vi "Scan Registry for USB Device.vi"() -> ()   [LabVIEW 2022 SP3]
uses:
  <vilib>/regexp/Match Regular Expression.xnode
panel:
  in  "error in (no error)":errorcluster
  out "error out":errorcluster
  in  "Device ID to Check if Present":string="051939001D4A1B03"
  out "Device Present?":bool
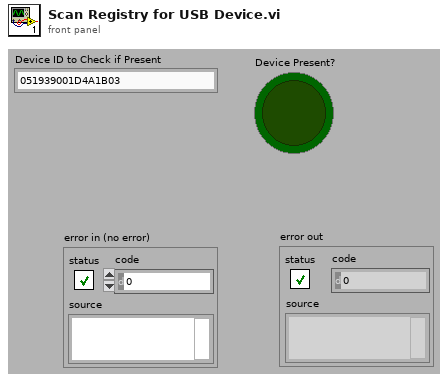
[diagram p1: front panel]
types:
  T1 = typedef "Registry refnum.ctl" = refnum<k1>
  T2 = cluster{"numValues":i32, "maxValueNameLen":i32, "maxValueDataLen":i32}
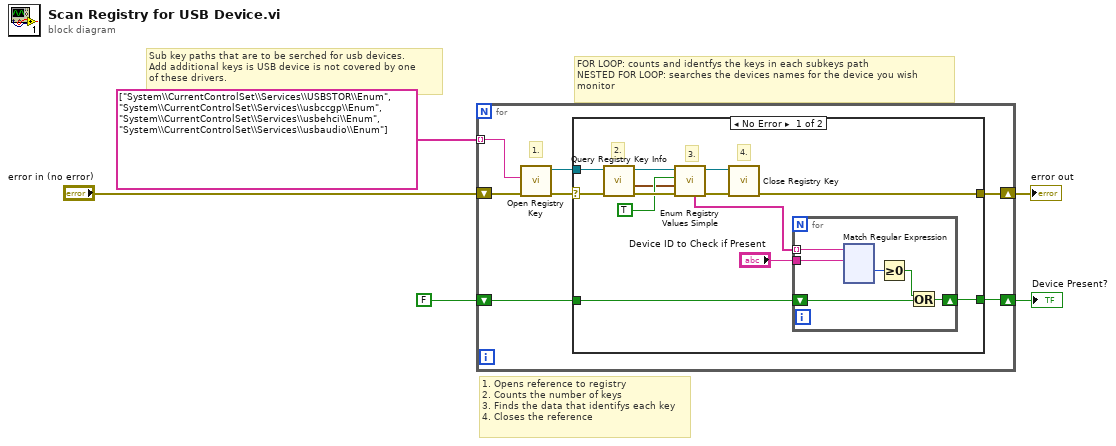
[diagram p0: block diagram]
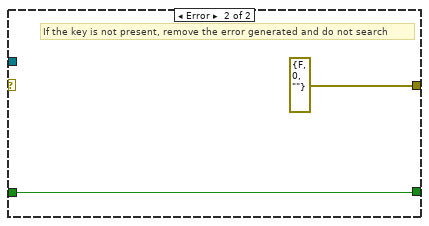
[diagram p2: hidden frame]
diagram:
  # "1. Opens reference to registry\n2. Counts the number of keys\n3. Finds the data that identifys each key\n4. Closes the reference"
  # "FOR LOOP: counts and identfys the keys in each subkeys path\nNESTED FOR LOOP: searches the devices names for the device you wish\nmonitor"
  # "Sub key paths that are to be serched for usb devices.\nAdd additional keys is USB device is not covered by one\nof these drivers."
  n1 = for {
    tunnel: string[] ["System\\CurrentControlSet\\Services\\USBSTOR\\Enum", "System\\CurrentControlSet\\Services\\usbccgp\\Enum", "System\\CurrentControlSet\\Services\\usbehci\\Enum", "System\\CurrentControlSet\\Services\\usbaudio\\Enum"] -> [w12] mode=indexing
    shift-right: [w8] -> w4
    shift-left: "error in (no error)" -> [w9]
    shift-right: [w6] -> w2
    shift-left: FALSE -> [w7]
    # "1."
    n2 = call <vilib>:"Open Registry Key.vi"("error in (no error)"=w9, "subkey"=w12) -> ("error out"=w11:errorcluster, "refnum out"=w10:T1)  [unwired: 1 in, 7 out]
    n3 = case shown="No Error" w11 {
      selector: w11 -> [w16 _]
      tunnel: w10 -> [w17 _]
      tunnel: [w15 errorcluster {"status"=FALSE, "code"=0, "source"=""} ("error in (no error)")] -> w8
      tunnel: w7 -> [w14 w149]
      tunnel: [w13 w149] -> w6
      frame No Error {
        # "4."
        # "3."
        # "2."
        n4 = call <vilib>:"Query Registry Key Info.vi"("error in (no error)"=w16, "refnum"=w17) -> ("error out"=w25:errorcluster, "value info"=w18:T2, "refnum out"=w24:T1)  [unwired: 7 out]
        n5 = call <vilib>:"Enum Registry Values Simple.vi"("error in (no error)"=w25, "value info"=w18, "retrieve data? (F)"=TRUE, "refnum"=w24) -> ("error out"=w20:errorcluster, "refnum out"=w19:T1, "String/Binary data"=w21:string[])  [unwired: 5 out]
        n6 = call <vilib>:"Close Registry Key.vi"("error in (no error)"=w20, "refnum"=w19) -> ("error out"=w15:errorcluster)  [unwired: 5 out]
        n7 = for {
          tunnel: "Device ID to Check if Present" -> [w31]
          tunnel: w21 -> [w30] mode=indexing
          shift-right: [w26] -> w13
          shift-left: w14 -> [w29]
          n8 = xnode "Match Regular Expression"("input string"=w30, "regular expression"=w31) -> ("offset past match"=w28:i32)  [unwired: 2 in, 6 out]
          n9 = Greater Or Equal To 0?(x=w28) -> (x >= 0?=w27:bool)
          n10 = Or(x=w27, y=w29) -> (x .or. y?=w26:bool)
        }
      }
      frame Error {
        # "If the key is not present, remove the error generated and do not search"
      }
    }
  }
  "error out" <- w4
  "Device Present?" <- w2
